vi "Open VISA Resource.vi"(7 "start path":path, 8 "error in (no error)":errorcluster, 9 "Modbus Address":u16=1 min=1 max=255 step=1, 10 "IP Address":string, 11 "heater_parent in":refnum<class "heater_parent.lvclass">) -> (0 "error out":errorcluster, 2 "Comms Failure":bool, 3 "heater_parent out":refnum<class "heater_parent.lvclass">)   [LabVIEW 2020, in "polar_bear_plus_drivers.lvlib" / "heater_parent.lvclass"]
uses:
  <instrlib>/RxnRover/Driver Polar Bear Plus/heater_parent/heater_parent.lvclass
  <instrlib>/RxnRover/Driver Polar Bear Plus/heater_parent/heater_parent.lvclass/heater_parent.ctl
  <instrlib>/Eurotherm nanodac/Eurotherm nanodac.lvlib
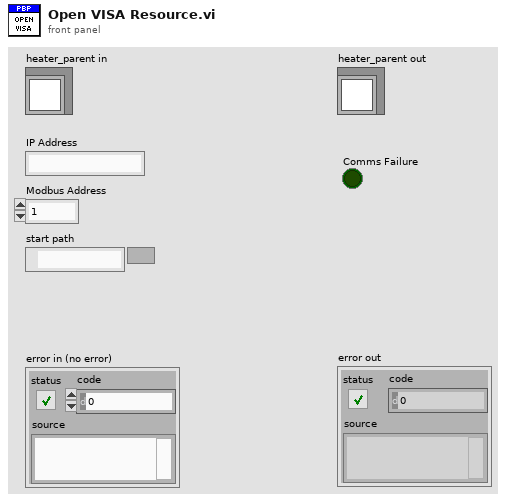
[diagram p1: front panel]
types:
  T1 = typedef "Eurotherm nanodac.lvlib/Parameter Info.ctl" = cluster{"Reference Name":string, "Modbus Address":u16, "Bisynch Mnemonic":string, "Data Type":enum16{"BOOL", "STATE_T", "UINT8", "INT16", "UINT16", "INT32", "UINT32", "TIME_T", "MODBUS_ADDRESS", "FLOAT32", "32BYTES", "EFLOAT32", "ETIME_T", "EINT32", "STRING_T"}, "Availability":string, "Alterability":string, "Low Limit":string, "High Limit":string, "Storage Type":enum16{"RAM", "NON-VOL"}, "Display Resolution":enum16{"0", "1", "2", "PV", "N/A"}, "User Access Conf":enum16{"ALTR", "READ", "HIDE", "N/A"}, "Factory Comms Address":u16, "Enumeration List":string, "Bit Mask":u16, "Description":string}
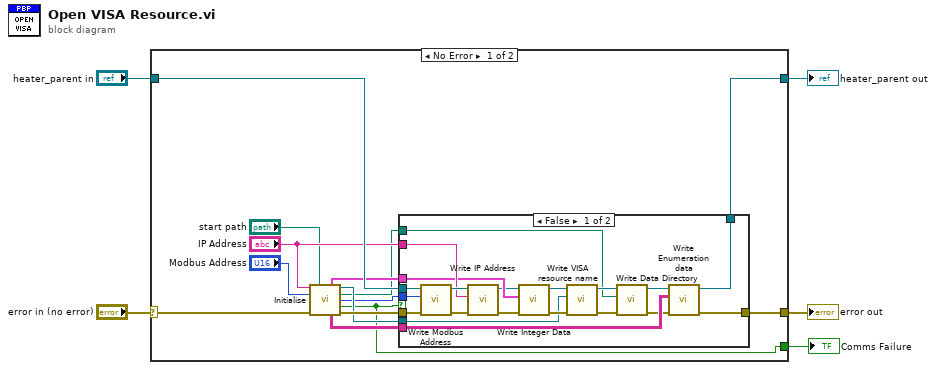
[diagram p0: block diagram]
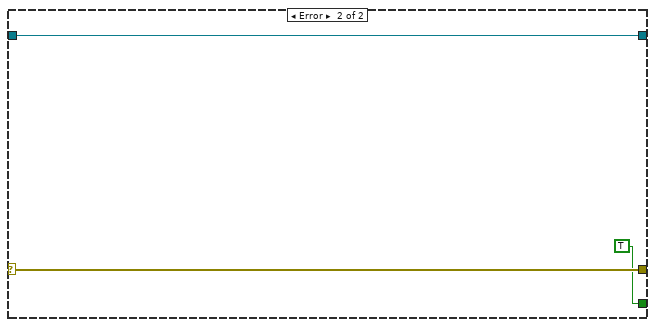
[diagram p3: hidden frame]
diagram:
  n1 = case shown="No Error" "error in (no error)" {
    selector: "error in (no error)" -> [w18 w44]
    tunnel: [w14 w44] -> w5
    tunnel: "heater_parent in" -> [w17 w43]
    tunnel: [w12 w43] -> w2
    tunnel: [w11 TRUE] -> w1
    frame No Error {
      n2 = call <instrlib>:"Initialise.vi"("IP Address"="IP Address", "start path"="start path", "Modbus Address"="Modbus Address", "error in (no error)"=w18) -> ("Integer Data"=w16:T1[], "VISA resource name out"=w15:refnum<visa-resource-name>, "Data Directory out"=w7:path, "Modbus Address Out"=w6:u8, "Comms Failure (F: OK)"=w11:bool, "Enumeration data"=w13:string[][], "error out"=w19:errorcluster)  [unwired: 5 in]
      n3 = case shown="False" w11 {
        tunnel: w19 -> [w39 w40]
        tunnel: w17 -> [w35 w41]
        tunnel: w6 -> [w32 _]
        tunnel: "IP Address" -> [w31 _]
        tunnel: w16 -> [w30 _]
        tunnel: w15 -> [w27 _]
        tunnel: [w26 w40] -> w14
        tunnel: w13 -> [w25 _]
        tunnel: [w24 w41] -> w12
        tunnel: w7 -> [w20 _]
        frame False {
          n4 = call-dynamic "Write Modbus Address.vi"("error in (no error)"=w39, "Modbus Address"=w32, "heater_parent in"=w35) -> ("error out"=w38:errorcluster, "heater_parent out"=w36:refnum<class "heater_parent.lvclass">)  [unwired: 7 in]
          n5 = call-dynamic "Write IP Address.vi"("error in (no error)"=w38, "IP Address"=w31, "heater_parent in"=w36) -> ("error out"=w37:errorcluster, "heater_parent out"=w29:refnum<class "heater_parent.lvclass">)  [unwired: 7 in]
          n6 = call-dynamic "Write Integer Data.vi"("error in (no error)"=w37, "Integer Data"=w30, "heater_parent in"=w29) -> ("error out"=w34:errorcluster, "heater_parent out"=w28:refnum<class "heater_parent.lvclass">)  [unwired: 7 in]
          n7 = call-dynamic "Write VISA resource name.vi"("error in (no error)"=w34, "VISA resource name"=w27, "heater_parent in"=w28) -> ("error out"=w33:errorcluster, "heater_parent out"=w22:refnum<class "heater_parent.lvclass">)  [unwired: 7 in]
          n8 = call-dynamic "Write Data Directory.vi"("error in (no error)"=w33, "Data Directory"=w20, "heater_parent in"=w22) -> ("error out"=w23:errorcluster, "heater_parent out"=w21:refnum<class "heater_parent.lvclass">)  [unwired: 7 in]
          n9 = call-dynamic "Write Enumeration data.vi"("error in (no error)"=w23, "Enumeration data"=w25, "heater_parent in"=w21) -> ("error out"=w26:errorcluster, "heater_parent out"=w24:refnum<class "heater_parent.lvclass">)  [unwired: 7 in]
        }
        frame True {
        }
      }
    }
    frame Error {
    }
  }
  "error out" <- w5
  "heater_parent out" <- w2
  "Comms Failure" <- w1
